vi "IStageClose.vi"(1 "PRIORLib.IStage":refnum<k7>) -> (0 "error out":errorcluster)   [LabVIEW 2011]
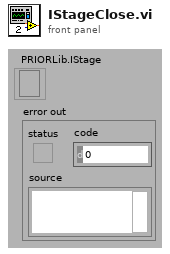
[diagram p1: front panel]
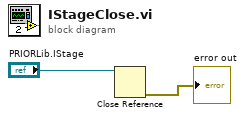
[diagram p0: block diagram]
diagram:
  n1 = Close Reference(reference="PRIORLib.IStage") -> (error out=→"error out":errorcluster)  [unwired: 1 in]
